vi "Random_passive.vi"(9 "Degree Max.":u16=15 min=1, 10 "Total trial":u16=30 min=1, 11 "Test mode\n(Simple or AXB paradigm)?":bool) -> (0 "Extreme":i8[](array[numeric]), 1 "Total Trial out":u16=30 caption="Number of Trials", 2 "Target":dbl[](array[numeric]), 3 "Target Type":bool[](array[boolean]))   [LabVIEW 2012]
uses:
  <vilib>/Analysis/1siggen.llb/Riffle Array (I32).vi
  <vilib>/Analysis/NI_AALBase.lvlib
panel:
  out "XY Graph":cluster{"Y":dbl[], "Y":dbl[]}[](graph)
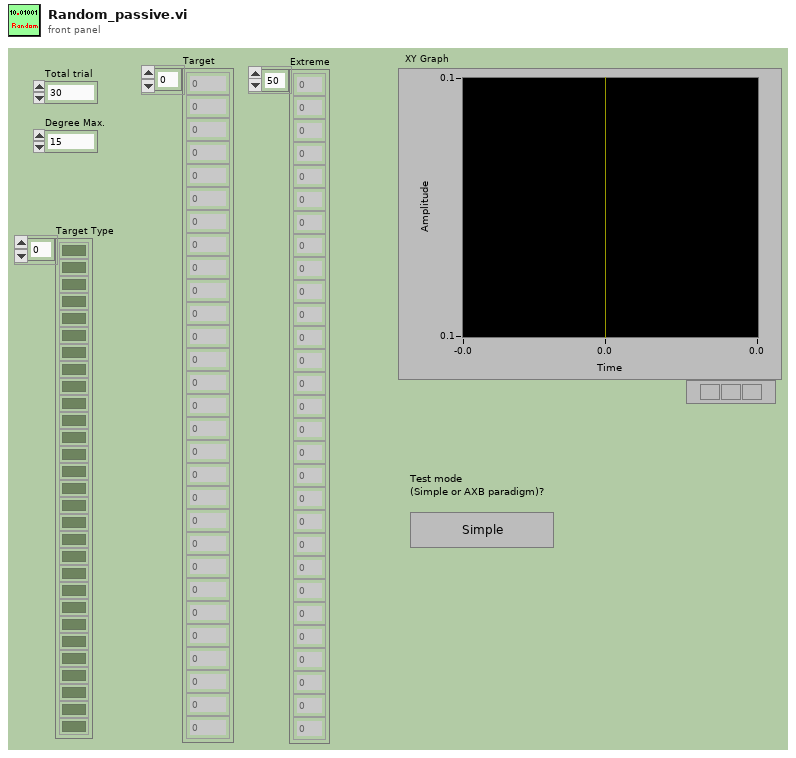
[diagram p1: front panel]
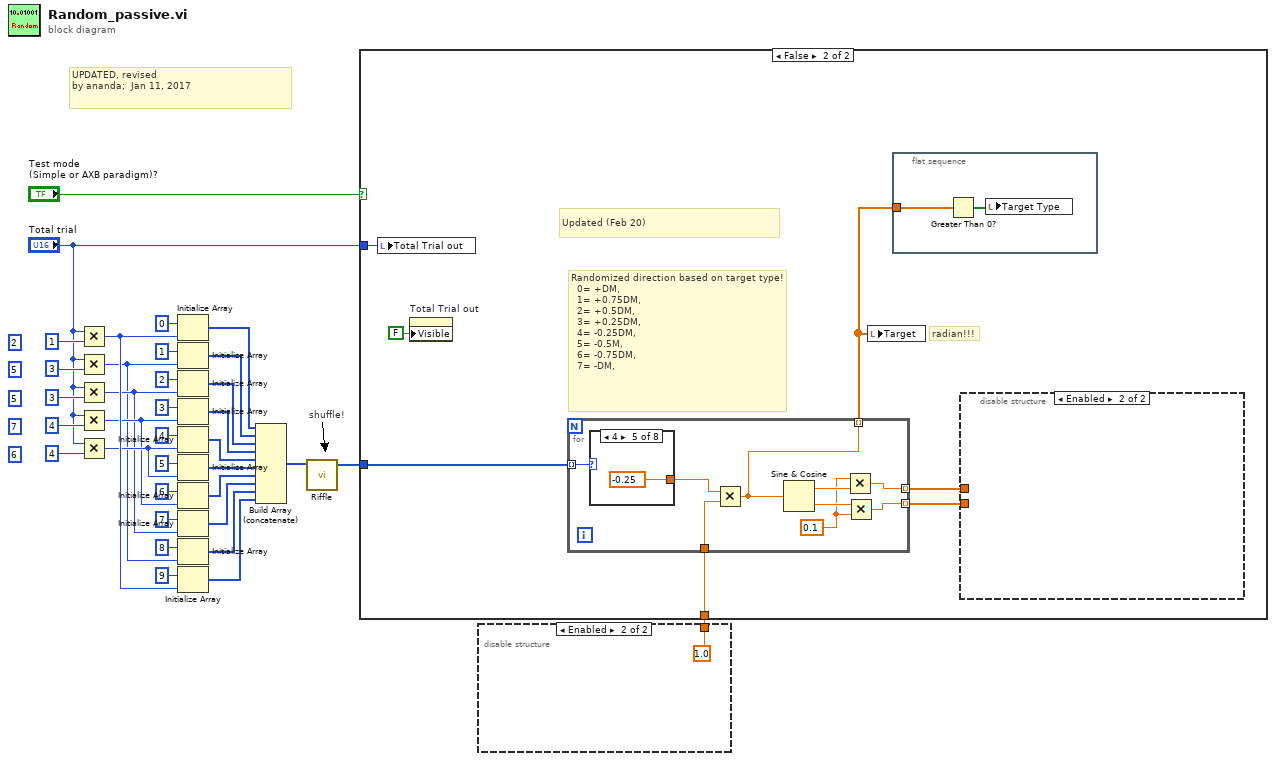
[diagram p0: block diagram]
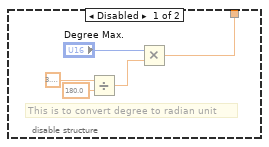
[diagram p2: hidden frame]
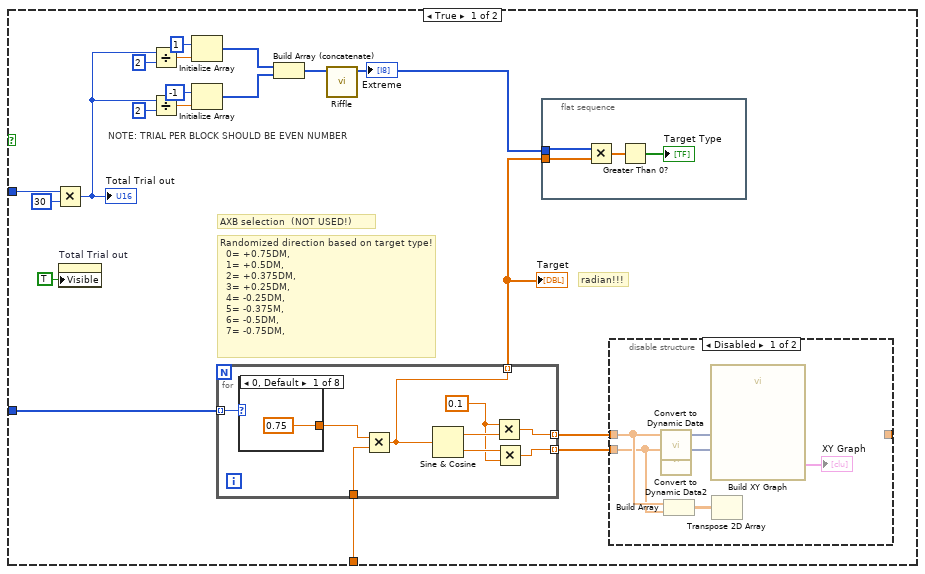
[diagram p3: hidden frame]
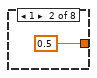
[diagram p5: hidden frame]
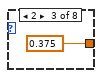
[diagram p6: hidden frame]
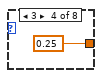
[diagram p7: hidden frame]
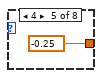
[diagram p8: hidden frame]
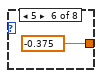
[diagram p9: hidden frame]
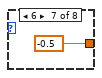
[diagram p10: hidden frame]
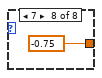
[diagram p11: hidden frame]
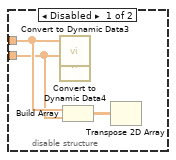
[diagram p12: hidden frame]
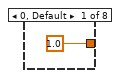
[diagram p13: hidden frame]
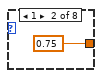
[diagram p14: hidden frame]
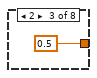
[diagram p15: hidden frame]
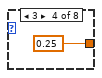
[diagram p16: hidden frame]
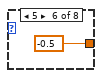
[diagram p17: hidden frame]
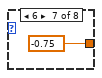
[diagram p18: hidden frame]
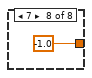
[diagram p19: hidden frame]
diagram:
  (unwired) u8 6 ("y")
  (unwired) u8 7 ("y")
  (unwired) u8 5 ("y")
  (unwired) u8 5 ("y")
  (unwired) u8 2 ("y")
  # "shuffle!"
  # "UPDATED, revised \nby ananda;  Jan 11, 2017"
  n1 = Multiply(x="Total trial", y=u8 1) -> (x*y=w10:u16)
  n2 = Multiply(x="Total trial", y=u8 3) -> (x*y=w4:u16)
  n3 = Multiply(x="Total trial", y=u8 3) -> (x*y=w5:u16)
  n4 = Multiply(x="Total trial", y=u8 4) -> (x*y=w6:u16)
  n5 = Multiply(x="Total trial", y=u8 4) -> (x*y=w7:u16)
  n6 = Initialize Array(u8 0 ("element"), w10) -> (w35:u8[])
  n7 = Initialize Array(u8 1 ("element"), w4) -> (w34:u8[])
  n8 = Initialize Array(u8 2 ("element"), w5) -> (w33:u8[])
  n9 = Initialize Array(u8 3 ("element"), w6) -> (w23:u8[])
  n10 = Initialize Array(u8 4 ("element"), w7) -> (w22:u8[])
  n11 = Initialize Array(u8 5 ("element"), w7) -> (w21:u8[])
  n12 = Initialize Array(u8 6 ("element"), w6) -> (w20:u8[])
  n13 = Initialize Array(u8 7 ("element"), w5) -> (w19:u8[])
  n14 = Initialize Array(u8 8 ("element"), w4) -> (w17:u8[])
  n15 = Initialize Array(u8 9 ("element"), w10) -> (w15:u8[])
  n16 = Build Array (concatenate)(w35, w34, w33, w23, w22, w21, w20, w19, w17, w15) -> (w29:u8[])
  n17 = call-poly <vilib>:"Riffle.vi"("X"=w29) -> ("Riffled {X}"=w3:i32[])  [unwired: 8 in, 2 out]
  n18 = disable-structure shown="Enabled" {
    disable-tunnel: [w36 1.0] -> w1
    frame Disabled {
      # "This is to convert degree to radian unit"
      n19 = Divide(x=3.141592653589793, y=180.0) -> (x/y=w39:dbl)
      n20 = Multiply(x="Degree Max.", y=w39) -> (x*y=w36:dbl)
    }
    frame Enabled {
    }
  }
  n21 = case shown="False" "Test mode\n(Simple or AXB paradigm)?" {
    tunnel: "Total trial" -> [w60 w91]
    tunnel: w3 -> [w59 w95]
    tunnel: w1 -> [w43 w92]
    frame True {
      # "radian!!!"
      # "NOTE: TRIAL PER BLOCK SHOULD BE EVEN NUMBER"
      # "AXB selection  (NOT USED!)"
      # "Randomized direction based on target type!\n  0= +0.75DM, \n  1= +0.5DM, \n  2= +0.375DM, \n  3= +0.25DM,\n  4= -0.25DM,\n  5= -0.375M,\n  6= -0.5DM,\n  7= -0.75DM,"
      n22 = Multiply(x=w60, y=u8 30) -> (x*y=w44:u16)
      "Total Trial out" <- w44
      n23 = property on="Total Trial out" class="DigNum (strict)"("Visible"=TRUE) -> ()  [unwired: 2 in, 2 out]
      n24 = Divide(x=w44, y=u8 2) -> (x/y=w56:dbl)
      n25 = Divide(x=w44, y=u8 2) -> (x/y=w51:dbl)
      n26 = Initialize Array(i8 1 ("element"), w56) -> (w49:i8[])
      n27 = Initialize Array(i8 -1 ("element"), w51) -> (w48:i8[])
      n28 = for {
        tunnel: w59 -> [w80] mode=indexing
        tunnel: w43 -> [w78]
        tunnel: [w76] -> w58 mode=indexing
        tunnel: [w74] -> w57 mode=indexing
        tunnel: [w72] -> w45 mode=indexing
        w73 = 0.1 ("y")
        n29 = case shown="0, Default" w80 {
          tunnel: [0.75 ("y") 0.5 ("y") 0.375 ("y") 0.25 ("y") -0.25 ("y") -0.375 ("y") -0.5 ("y") -0.75 ("y")] -> w79
          frame 0, Default {
          }
          frame 1 {
          }
          frame 2 {
          }
          frame 3 {
          }
          frame 4 {
          }
          frame 5 {
          }
          frame 6 {
          }
          frame 7 {
          }
        }
        n30 = Multiply(x=w79, y=w78) -> (x*y=w72:dbl)
        n31 = Sine & Cosine(0:w72) -> (1:w75:dbl, 2:w77:dbl)
        n32 = Multiply(x=w73, y=w75) -> (x*y=w76:dbl)
        n33 = Multiply(x=w77, y=w73) -> (x*y=w74:dbl)
      }
      "Target" <- w45
      n34 = Build Array (concatenate)(w49, w48) -> (w47:i8[])
      n35 = call-poly <vilib>:"Riffle.vi"("X"=w47) -> ("Riffled {X}"=w46:i32[])  [unwired: 8 in, 2 out]
      "Extreme" <- w46
      n36 = flat-sequence {
        tunnel: w46 -> [w62]
        tunnel: w45 -> [w61]
        frame #0 {
          n37 = Multiply(x=w62, y=w61) -> (x*y=w64:dbl[])
          n38 = Greater Than 0?(x=w64) -> (x > 0?=→"Target Type":bool[])
        }
      }
      n39 = disable-structure shown="Disabled" {
        disable-tunnel: w58 -> [w69 w71]
        disable-tunnel: w57 -> [w68 _]
        disable-tunnel: [_ w71] -> _
        frame Disabled {
          n40 = call "Convert to Dynamic Data"("Array"=w69) -> ("Dynamic Data Type"=w66:dynamicdata)  [unwired: 3 in]
          n41 = call "Convert to Dynamic Data2"("Array"=w68) -> ("Dynamic Data Type"=w65:dynamicdata)  [unwired: 3 in]
          n42 = Build Array(w69, w68) -> (w70:dbl[][])
          n43 = call "Build XY Graph"("Y Input"=w65, "X Input"=w66) -> ("XY Graph"=→"XY Graph":cluster{"Y":dbl[], "Y":dbl[]}[])  [unwired: 3 in, 6 out]
          n44 = Transpose 2D Array(2D array=w70) -> ()  [unwired: 1 out]
        }
        frame Enabled {
        }
      }
    }
    frame False {
      # "Updated (Feb 20)"
      # "radian!!!"
      # "Randomized direction based on target type!\n  0= +DM, \n  1= +0.75DM, \n  2= +0.5DM, \n  3= +0.25DM,\n  4= -0.25DM,\n  5= -0.5M,\n  6= -0.75DM,\n  7= -DM,"
      n45 = local write "Total Trial out"(w91) -> ()
      n46 = property on="Total Trial out" class="DigNum (strict)"("Visible"=FALSE) -> ()  [unwired: 2 in, 2 out]
      n47 = for {
        tunnel: w95 -> [w109] mode=indexing
        tunnel: w92 -> [w107]
        tunnel: [w105] -> w94 mode=indexing
        tunnel: [w103] -> w93 mode=indexing
        tunnel: [w101] -> w89 mode=indexing
        w102 = 0.1 ("y")
        n48 = case shown="4" w109 {
          tunnel: [1.0 ("y") 0.75 ("y") 0.5 ("y") 0.25 ("y") -0.25 ("y") -0.5 ("y") -0.75 ("y") -1.0 ("y")] -> w108
          frame 0, Default {
          }
          frame 1 {
          }
          frame 2 {
          }
          frame 3 {
          }
          frame 4 {
          }
          frame 5 {
          }
          frame 6 {
          }
          frame 7 {
          }
        }
        n49 = Multiply(x=w108, y=w107) -> (x*y=w101:dbl)
        n50 = Sine & Cosine(0:w101) -> (1:w104:dbl, 2:w106:dbl)
        n51 = Multiply(x=w102, y=w104) -> (x*y=w105:dbl)
        n52 = Multiply(x=w106, y=w102) -> (x*y=w103:dbl)
      }
      n53 = local write "Target"(w89) -> ()
      n54 = flat-sequence {
        tunnel: w89 -> [w97]
        frame #0 {
          n55 = Greater Than 0?(x=w97) -> (x > 0?=w96:bool[])
          n56 = local write "Target Type"(w96) -> ()
        }
      }
      n57 = disable-structure shown="Enabled" {
        disable-tunnel: w94 -> [w99 _]
        disable-tunnel: w93 -> [w98 _]
        frame Disabled {
          n58 = call "Convert to Dynamic Data3"("Array"=w99) -> ()  [unwired: 3 in, 1 out]
          n59 = call "Convert to Dynamic Data4"("Array"=w98) -> ()  [unwired: 3 in, 1 out]
          n60 = Build Array(w99, w98) -> (w100:dbl[][])
          n61 = Transpose 2D Array(2D array=w100) -> ()  [unwired: 1 out]
        }
        frame Enabled {
        }
      }
    }
  }
